vi "matriz de leds.vi"() -> ()   [LabVIEW 2016]
panel:
  out "Array":bool[][](array[boolean])
  in  "Horizontal Pointer Slide":dbl(slide) scale=0.0..255.0
  out "new picture 2":picture
  out "new picture":picture
  in  "File Path Control":path
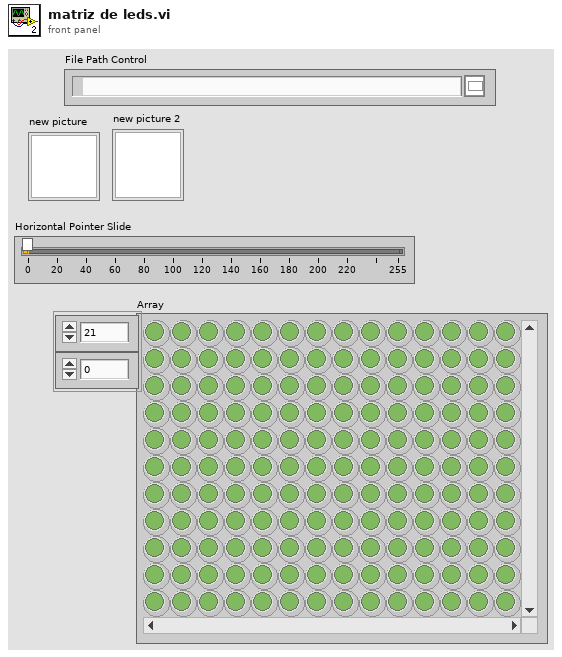
[diagram p1: front panel]
types:
  T1 = typedef "imagedata.ctl" = cluster{"image type":i32, "image depth":i32, "image":u8[], "mask":u8[], "colors":u32[], "Rectangle":cluster{"left":i16, "top":i16, "right":i16, "bottom":i16}}
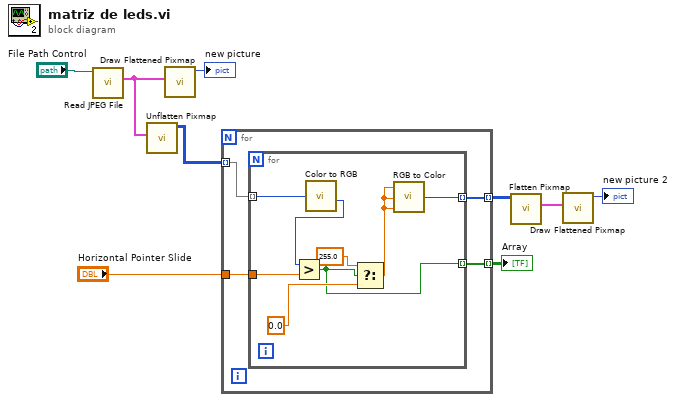
[diagram p0: block diagram]
diagram:
  n1 = call <vilib>:"Read JPEG File.vi"("path to JPEG file"="File Path Control") -> ("image data"=w7:T1)  [unwired: 8 in, 2 out]
  n2 = call <vilib>:"Unflatten Pixmap.vi"("image data"=w7) -> ("24-bit pixmap"=w6:u32[][])  [unwired: 4 in, 6 out]
  n3 = call <vilib>:"Draw Flattened Pixmap.vi"("image data"=w7) -> ("new picture"=→"new picture":picture)  [unwired: 8 in]
  n4 = for {
    tunnel: w6 -> [w13] mode=indexing
    tunnel: [w12] -> w5 mode=indexing
    tunnel: "Horizontal Pointer Slide" -> [w11]
    tunnel: [w10] -> w1 mode=indexing
    n5 = for {
      tunnel: w13 -> [w21] mode=indexing
      tunnel: [w20] -> w12 mode=indexing
      tunnel: w11 -> [w16]
      tunnel: [w14] -> w10 mode=indexing
      n6 = call <vilib>:"Color to RGB.vi"("Color"=w21) -> ("G"=w15:u8)  [unwired: 3 out]
      n7 = Greater?(x=w15, y=w16) -> (0:w14:bool)
      n8 = Select(t=255.0, s=w14, f=0.0) -> (s? t:f=w17:dbl)
      n9 = call <vilib>:"RGB to Color.vi"("B"=w17, "G"=w17, "R"=w17) -> ("Color"=w20:u32)
    }
  }
  "Array" <- w1
  n10 = call <vilib>:"Flatten Pixmap.vi"("24-bit pixmap"=w5) -> ("image data"=w4:T1)  [unwired: 10 in]
  n11 = call <vilib>:"Draw Flattened Pixmap.vi"("image data"=w4) -> ("new picture"=→"new picture 2":picture)  [unwired: 8 in]
